vi "HandleWash.vi"(7 "Vehicle Position":T2, 9 "Message Queue Data":T3, 10 "Command":T1, 11 "queue in":refnum<queue>) -> (2 "Time Remaining":u32, 3 "car wash indicators":T4)   [LabVIEW 2018]
uses:
  MessageQueueData.ctl
  Command.ctl
  Position.ctl
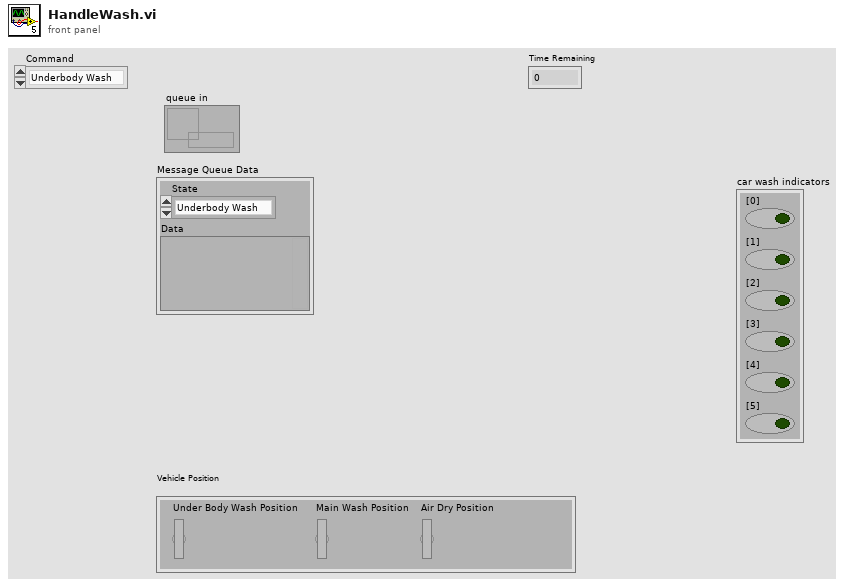
[diagram p1: front panel]
types:
  T1 = typedef "Command.ctl" = enum16{"Underbody Wash", "Soap Application", "Main High-Pressure Wash", "Clear Water Rinse", "Air Dry Cycle", "Stop"}
  T2 = typedef "Position.ctl" = enum32{"Under Body Wash Position", "Main Wash Position", "Air Dry Position"}
  T3 = typedef "MessageQueueData.ctl" = cluster{"State":T1, "Data":variant}
  T4 = cluster{"[0]":bool, "[1]":bool, "[2]":bool, "[3]":bool, "[4]":bool, "[5]":bool}
  T5 = typedef "WashState.ctl" = cluster{"Time Remaining":i32, "LastTickCount":i32, "Required Vehicle Position":T2}
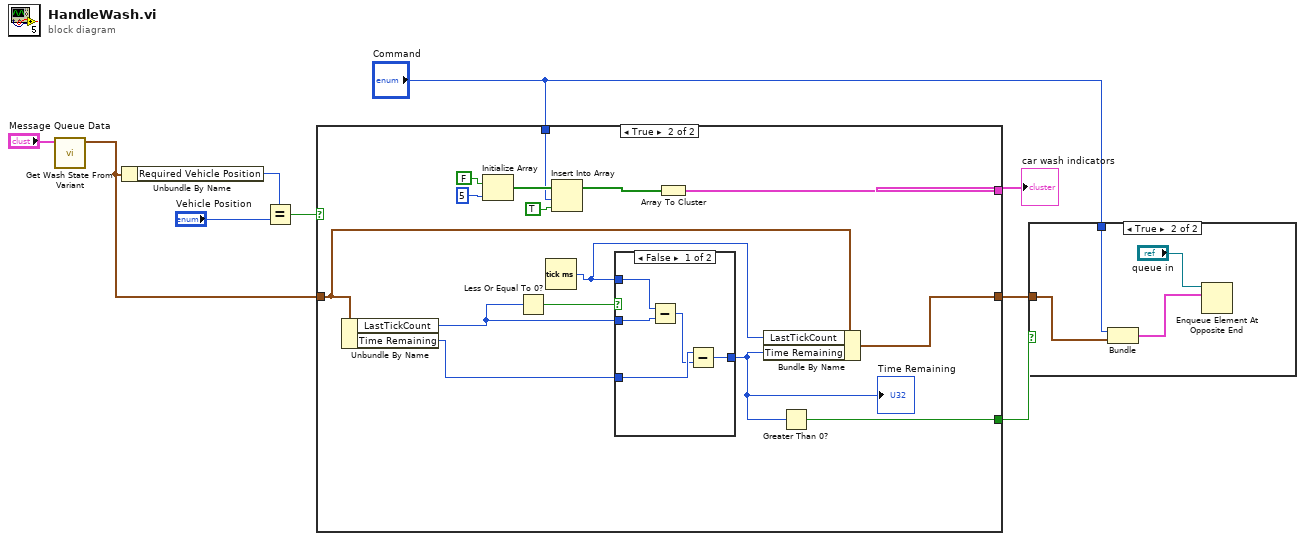
[diagram p0: block diagram]
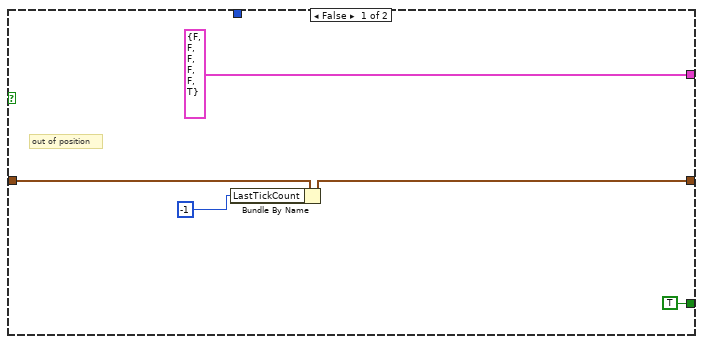
[diagram p3: hidden frame]
diagram:
  n1 = call "Get Wash State From Variant.vi"("Message Queue Data"="Message Queue Data") -> ("WashState out"=w3:T5)  [unwired: 9 in, 1 out]
  n2 = Unbundle By Name(w3) -> ("Required Vehicle Position"=w9:T2)
  n3 = Equal?(x=w9, y="Vehicle Position") -> (x = y?=w7:bool)
  n4 = case shown="True" w7 {
    tunnel: [T4 {"[0]"=FALSE, "[1]"=FALSE, "[2]"=FALSE, "[3]"=FALSE, "[4]"=FALSE, "[5]"=TRUE} w24] -> w6
    tunnel: w3 -> [w13 w22]
    tunnel: [w12 w21] -> w5
    tunnel: [TRUE w16] -> w4
    tunnel: "Command" -> [_ w15]
    frame False {
      # "out of position"
      n5 = Bundle By Name(cluster=w13, "LastTickCount"=-1 ("StartTime")) -> (w12:T5)
    }
    frame True {
      n6 = Unbundle By Name(w22) -> ("LastTickCount"=w20:i32, "Time Remaining"=w19:i32)
      n7 = Initialize Array(FALSE ("Air Dry"), 5 ("dimension size")) -> (w27:bool[])
      n8 = Less Or Equal To 0?(x=w20) -> (x <= 0?=w23:bool)
      n9 = Tick Count (ms)() -> (millisecond timer value=w18:u32)
      n10 = Insert Into Array(array=w27, index=w15, new element=TRUE ("new element/subarray")) -> (w29:bool[])
      n11 = case shown="False" w23 {
        tunnel: w18 -> [w34 _]
        tunnel: w20 -> [w33 _]
        tunnel: w19 -> [w32 w35]
        tunnel: [w30 w35] -> w17
        frame False {
          n12 = Subtract(x=w34, y=w33) -> (x-y=w31:u32)
          n13 = Subtract(x=w32, y=w31) -> (x-y=w30:u32)
        }
        frame True {
        }
      }
      "Time Remaining" <- w17
      n14 = Array To Cluster(array=w29) -> (cluster=w24:T4)
      n15 = Bundle By Name(cluster=w22, "LastTickCount"=w18, "Time Remaining"=w17) -> (w21:T5)
      n16 = Greater Than 0?(x=w17) -> (x > 0?=w16:bool)
    }
  }
  "car wash indicators" <- w6
  n17 = case shown="True" w4 {
    tunnel: w5 -> [_ w37]
    tunnel: "Command" -> [_ w38]
    frame False {
    }
    frame True {
      n18 = Bundle("Command"=w38, "WashState out"=w37) -> (w36:cluster{"Command":T1, "WashState out":T5})  [unwired: 1 in]
      n19 = Enqueue Element At Opposite End(queue="queue in", element=w36) -> ()  [unwired: 2 in, 3 out]
    }
  }
